vi "Begin.vi"(8 "error in":errorcluster) -> (0 "error out":errorcluster)   [LabVIEW 2014]
doc: "Called before other user functions, this VI is expected to open initial I/O refnums, load in file data, and do all program initialization. Notice that the <B>error out</B> terminal is simply used for data flow. Wiring it to other structures or subVIs ensures that this VI runs first."
uses:
  <vilib>/Rock Robotics/SystemInterfaces/DIO/FPGA_DIOPWMChannel.ctl
  <vilib>/Rock Robotics/WPI/SafetyOutput/WPI_SafetyOutputConfigMenu.ctl
  <vilib>/Rock Robotics/WPI/DriverStation/WPI_DriverStationRobotMode2.ctl
  <vilib>/Rock Robotics/WPI/Joystick/WPI_JoystickDeviceEnum.ctl
  <vilib>/Rock Robotics/WPI/CAN/Jaguar/SubVIs/WPI_CANJaguar_ControlMode.ctl
  <vilib>/Rock Robotics/WPI/CAN/Jaguar/SubVIs/WPI_CANJaguar_PositionReference.ctl
  <vilib>/Rock Robotics/WPI/CAN/Jaguar/SubVIs/WPI_CANJaguar_LimitMode.ctl
  <vilib>/Rock Robotics/WPI/CAN/Jaguar/SubVIs/WPI_CANJaguar_BrakeCoastMode.ctl
  <vilib>/Rock Robotics/WPI/RobotDrive/WPI_RobotDriveOpen2MotorWithTalon.vi
  Robot Global Data.vi
  <vilib>/Rock Robotics/Network Tables/SD Write String Array.vi
  <vilib>/Rock Robotics/WPI/MotorControl/WPI_MotorControlOpenCANJaguar.vi
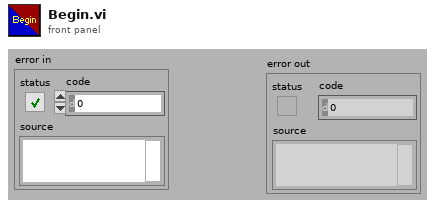
[diagram p1: front panel]
types:
  T1 = typedef "WPI_CANJaguar_BrakeCoastMode.ctl" = enum8{"Jumper", "Brake", "Coast"}
  T2 = typedef "WPI_CANJaguar_LimitMode.ctl" = enum16{"Switch Inputs Only", "Soft Position Limits"}
  T3 = typedef "WPI_CANJaguar_PositionReference.ctl" = u8
  T4 = typedef "WPI_CANJaguar_ControlMode.ctl" = enum8{"Percent VBus", "Current", "Speed", "Position", "Voltage"}
  T5 = typedef "WPI_JoystickDeviceEnum.ctl" = enum16{"USB 0", "USB 1", "USB 2", "USB 3", "USB 4", "USB 5"}
  T6 = typedef "WPI_DriverStationRobotMode2.ctl" = enum16{"Autonomous Disabled", "Autonomous Enabled", "Teleop Disabled", "Teleop Enabled", "Disconnected", "Finish", "Test Disabled", "Test Enabled", "Emergency Stopped"}
  T7 = typedef "WPI_SafetyOutputConfigMenu.ctl" = enum16{"Enable", "Disable"}
  T8 = typedef "FPGA_DIOPWMChannel.ctl" = enum8{"PWM 0", "PWM 1", "PWM 2", "PWM 3", "PWM 4", "PWM 5", "PWM 6", "PWM 7", "PWM 8", "PWM 9", "PWM MXP 0", "PWM MXP 1", "PWM MXP 2", "PWM MXP 3", "PWM MXP 4", "PWM MXP 5", "PWM MXP 6", "PWM MXP 7", "PWM MXP 8", "PWM MXP 9", "Invalid"}
  T9 = typedef "WPI_JoystickDevRef.ctl" = cluster{"Device":T5}
  T10 = typedef "WPI_RobotDriveDevRef.ctl" = cluster{"DevStatus":errorcluster, "Motors[]":T11[], "Square Inputs":bool, "Max Output":dbl}
  T11 = typedef "WPI_MotorControlDeviceRef.ctl" = cluster{"DeviceStatus":errorcluster, "Type":T12, "PWM":cluster{"Controller":T13, "PWM Channel":T8, "DeadBand":T14}, "CAN":cluster{"Device Number":u8, "Control Mode":T4, "Semaphore":T15, "Max Vout":dbl, "TalonSRX Control Mode":T16}, "Invert":bool, "TransformRef":T17, "InvTransformRef":T17}
  T12 = typedef "WPI_MotorControlType.ctl" = enum16{"PWM", "CAN", "CANTalonSRX"}
  T13 = typedef "FPGA_TypedefDigitalModule.ctl" = enum16{"Controller 1"}
  T14 = typedef "WPI_PWMDeadband.ctl" = cluster{"Name":string, "maxPositivePwm":i32, "minPositivePwm":i32, "centerPwm":i32, "maxNegativePwm":i32, "minNegativePwm":i32, "angularRange":u16}
  T15 = typedef "Semaphore RefNum" = refnum<k1>
  T16 = typedef "WPI_CANTalonSRX_APIControlMode.ctl" = enum8{"Percent VBus", "Speed", "Position", "Slave", "Unchanged / Invalid"}
  T17 = typedef "WPI_PWMTransform_ConPane.ctl" = refnum<vi>
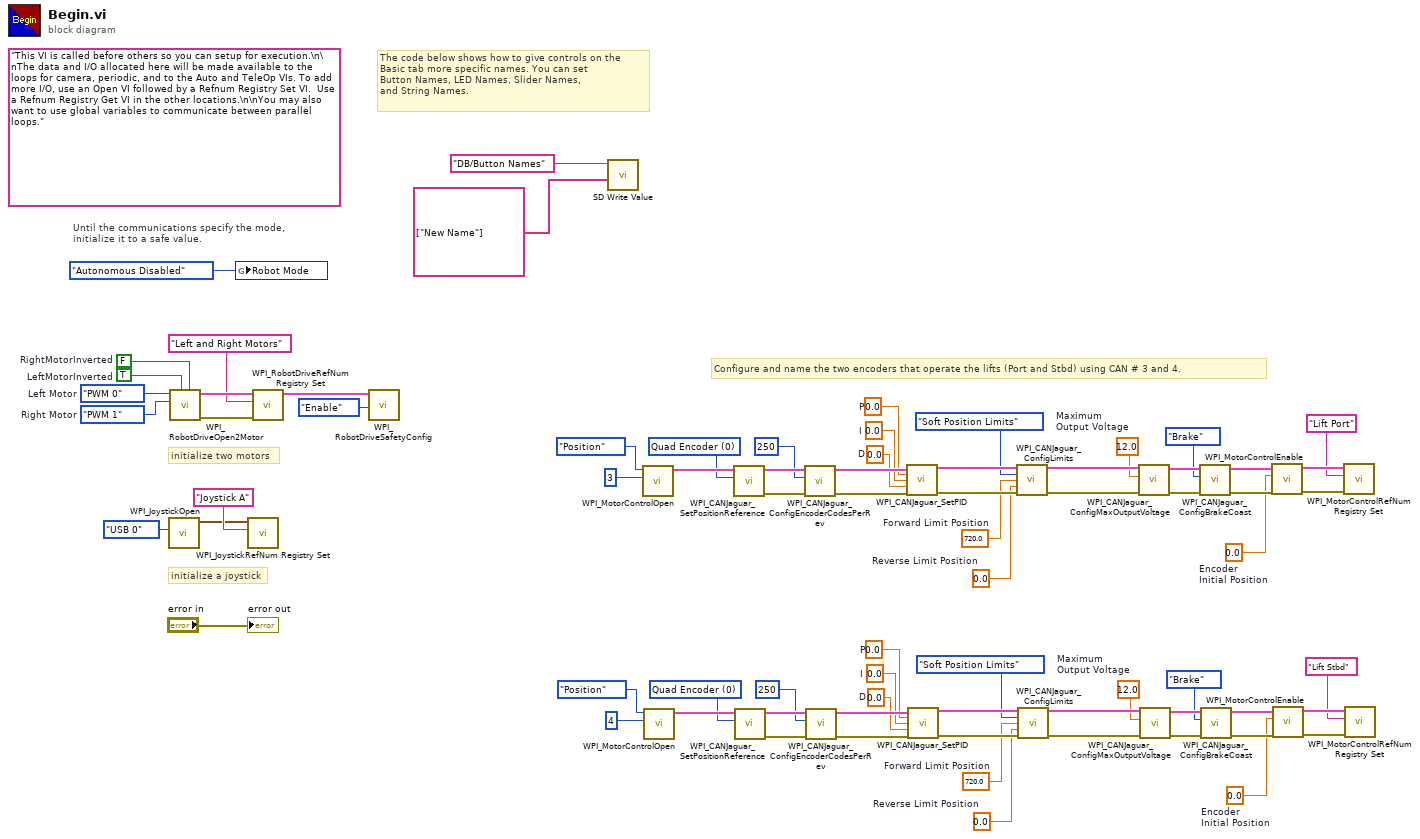
[diagram p0: block diagram]
diagram:
  w4 = 0.0  # Encoder  Initial Position
  w10 = 12.0  # Maximum  Output Voltage
  w13 = 0.0  # Reverse Limit Position
  w14 = 720.0  # Forward Limit Position
  w18 = 0.0  # D
  w19 = 0.0  # I
  w20 = 0.0  # P
  w26 = T3 0 items=["Quad Encoder"=0, "Potentiometer"=1, "None"=255] ("Position Reference")
  w33 = 0.0  # Encoder  Initial Position
  w39 = 12.0  # Maximum  Output Voltage
  w42 = 0.0  # Reverse Limit Position
  w43 = 720.0  # Forward Limit Position
  w47 = 0.0  # D
  w48 = 0.0  # I
  w49 = 0.0  # P
  w55 = T3 0 items=["Quad Encoder"=0, "Potentiometer"=1, "None"=255] ("Position Reference")
  (unwired) "This VI is called before others so you can setup for execution.\n\nThe data and I/O allocated here will be made available to the loops for camera, periodic, and to the Auto and TeleOp VIs. To add more I/O, use an Open VI followed by a Refnum Registry Set VI.  Use a Refnum Registry Get VI in the other locations.\n\nYou may also want to use global variables to communicate between parallel loops."
  w68 = FPGA_DIOPWMChannel."PWM 1"  # Right Motor
  w69 = FPGA_DIOPWMChannel."PWM 0"  # Left Motor
  w73 = TRUE  # LeftMotorInverted
  w74 = FALSE  # RightMotorInverted
  # "Configure and name the two encoders that operate the lifts (Port and Stbd) using CAN # 3 and 4."
  # "The code below shows how to give controls on the\nBasic tab more specific names. You can set\nButton Names, LED Names, Slider Names,\nand String Names."
  # "initialize a joystick"
  # "Until the communications specify the mode,\ninitialize it to a safe value."
  # "initialize two motors"
  n1 = call <vilib>:"WPI_JoystickOpen.vi"("JoystickDevice"=WPI_JoystickDeviceEnum."USB 0") -> ("JoystickDevRef"=w63:T9)  [unwired: 10 in]
  n2 = call-poly <vilib>:"WPI_RobotDriveOpen2Motor.vi"("Right Motor Inverted"=w74, "Left Motor Inverted"=w73, "Right Motor"=w68, "Left Motor"=w69) -> ("error out"=w70:errorcluster, "RobotDriveDevRef"=w72:T10)  [unwired: 1 in, 5 out]
  n3 = global write "Robot Global Data.vi" "Robot Mode"(WPI_DriverStationRobotMode2."Autonomous Disabled" ("Robot Mode")) -> ()
  n4 = call <vilib>:"WPI_JoystickRefNum Registry Set.vi"("refnum name"="Joystick A", "JoystickDevRef"=w63) -> ()  [unwired: 8 in, 2 out]
  n5 = call <vilib>:"WPI_RobotDriveRefNum Registry Set.vi"("error in (no error)"=w70, "refnum name"="Left and Right Motors", "RobotDriveDevRef"=w72) -> ("RobotDriveDevRef"=w67:T10)  [unwired: 8 out]
  n6 = call <vilib>:"WPI_RobotDriveSafetyConfig.vi"("mode"=WPI_SafetyOutputConfigMenu."Enable", "RobotDriveDevRef"=w67) -> ()  [unwired: 8 in, 2 out]
  n7 = call-poly <vilib>:"SD Write Value.vi"("String Array"=string[] ["New Name"], "Name"="DB/Button Names") -> ()  [unwired: 8 in, 2 out]
  n8 = call-poly <vilib>:"WPI_MotorControlOpen.vi"("Device Number"=u8 3, "Control Mode"=WPI_CANJaguar_ControlMode."Position") -> ("MotorControlDeviceRef"=w56:T11)  [unwired: 8 in, 1 out]
  n9 = call-poly <vilib>:"WPI_MotorControlOpen.vi"("Device Number"=u8 4, "Control Mode"=WPI_CANJaguar_ControlMode."Position") -> ("MotorControlDeviceRef"=w27:T11)  [unwired: 8 in, 1 out]
  n10 = call <vilib>:"WPI_CANJaguar_SetPositionReference.vi"("Position Reference"=w55, "CAN Jaguar Ref"=w56) -> ("error out"=w54:errorcluster, "CAN Jaguar Ref Out"=w53:T11)  [unwired: 8 in]
  n11 = call <vilib>:"WPI_CANJaguar_SetPositionReference.vi"("Position Reference"=w26, "CAN Jaguar Ref"=w27) -> ("error out"=w25:errorcluster, "CAN Jaguar Ref Out"=w24:T11)  [unwired: 8 in]
  n12 = call <vilib>:"WPI_CANJaguar_ConfigEncoderCodesPerRev.vi"("error in (no error)"=w54, "Encoder Codes Per Rev"=u16 250, "CAN Jaguar Ref"=w53) -> ("error out"=w50:errorcluster, "CAN Jaguar Ref Out"=w51:T11)  [unwired: 7 in]
  n13 = call <vilib>:"WPI_CANJaguar_ConfigEncoderCodesPerRev.vi"("error in (no error)"=w25, "Encoder Codes Per Rev"=u16 250, "CAN Jaguar Ref"=w24) -> ("error out"=w21:errorcluster, "CAN Jaguar Ref Out"=w22:T11)  [unwired: 7 in]
  n14 = call <vilib>:"WPI_CANJaguar_SetPID.vi"("CAN Jaguar Ref"=w51, "P"=w49, "I"=w48, "D"=w47, "error in (no error)"=w50) -> ("CAN Jaguar Ref Out"=w46:T11, "error out"=w45:errorcluster)  [unwired: 9 in]
  n15 = call <vilib>:"WPI_CANJaguar_SetPID.vi"("CAN Jaguar Ref"=w22, "P"=w20, "I"=w19, "D"=w18, "error in (no error)"=w21) -> ("CAN Jaguar Ref Out"=w17:T11, "error out"=w16:errorcluster)  [unwired: 9 in]
  n16 = call <vilib>:"WPI_CANJaguar_ConfigLimits.vi"("CAN Jaguar Ref"=w46, "Limit Mode"=WPI_CANJaguar_LimitMode."Soft Position Limits", "Forward Limit Position"=w43, "Reverse Limit Position"=w42, "error in (no error)"=w45) -> ("CAN Jaguar Ref Out"=w40:T11, "error out"=w41:errorcluster)  [unwired: 9 in]
  n17 = call <vilib>:"WPI_CANJaguar_ConfigLimits.vi"("CAN Jaguar Ref"=w17, "Limit Mode"=WPI_CANJaguar_LimitMode."Soft Position Limits", "Forward Limit Position"=w14, "Reverse Limit Position"=w13, "error in (no error)"=w16) -> ("CAN Jaguar Ref Out"=w11:T11, "error out"=w12:errorcluster)  [unwired: 9 in]
  n18 = call <vilib>:"WPI_CANJaguar_ConfigMaxOutputVoltage.vi"("error in (no error)"=w41, "Maximum Output Voltage"=w39, "CAN Jaguar Ref"=w40) -> ("error out"=w37:errorcluster, "CAN Jaguar Ref Out"=w38:T11)  [unwired: 7 in]
  n19 = call <vilib>:"WPI_CANJaguar_ConfigMaxOutputVoltage.vi"("error in (no error)"=w12, "Maximum Output Voltage"=w10, "CAN Jaguar Ref"=w11) -> ("error out"=w8:errorcluster, "CAN Jaguar Ref Out"=w9:T11)  [unwired: 7 in]
  n20 = call <vilib>:"WPI_CANJaguar_ConfigBrakeCoast.vi"("error in (no error)"=w37, "Brake / Coast Mode"=WPI_CANJaguar_BrakeCoastMode."Brake", "CAN Jaguar Ref"=w38) -> ("error out"=w35:errorcluster, "CAN Jaguar Ref Out"=w34:T11)  [unwired: 7 in]
  n21 = call <vilib>:"WPI_CANJaguar_ConfigBrakeCoast.vi"("error in (no error)"=w8, "Brake / Coast Mode"=WPI_CANJaguar_BrakeCoastMode."Brake", "CAN Jaguar Ref"=w9) -> ("error out"=w6:errorcluster, "CAN Jaguar Ref Out"=w5:T11)  [unwired: 7 in]
  n22 = call <vilib>:"WPI_MotorControlEnable.vi"("error in (no error)"=w35, "Encoder Initial Position"=w33, "CAN Jaguar Ref"=w34) -> ("error out"=w32:errorcluster, "CAN Jaguar Ref Out"=w31:T11)  [unwired: 7 in]
  n23 = call <vilib>:"WPI_MotorControlEnable.vi"("error in (no error)"=w6, "Encoder Initial Position"=w4, "CAN Jaguar Ref"=w5) -> ("error out"=w3:errorcluster, "CAN Jaguar Ref Out"=w2:T11)  [unwired: 7 in]
  n24 = call <vilib>:"WPI_MotorControlRefNum Registry Set.vi"("error in (no error)"=w32, "refnum name"="Lift Port", "MotorControlDevRef"=w31) -> ()  [unwired: 7 in, 2 out]
  n25 = call <vilib>:"WPI_MotorControlRefNum Registry Set.vi"("error in (no error)"=w3, "refnum name"="Lift Stbd", "MotorControlDevRef"=w2) -> ()  [unwired: 7 in, 2 out]
  "error out" <- "error in"
